vi "esdaq_init.vi"(0 "esdaqPortInp":refnum<visa-resource-name>) -> (1 "esdaqPortOut":refnum<visa-resource-name>, 2 "esdaqErrorOut":errorcluster)   [LabVIEW 2019]
uses:
  <vilib>/Instr/_visa.llb/VISA Flush IO Buffer Mask.ctl
  <vilib>/Instr/_visa.llb/VISA Configure Serial Port (Instr).vi
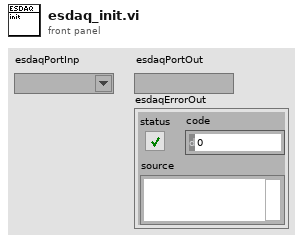
[diagram p1: front panel]
types:
  T1 = typedef "VISA Flush IO Buffer Mask.ctl" = u16
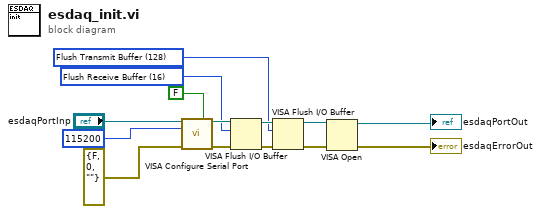
[diagram p0: block diagram]
diagram:
  w6 = T1 128 items=["Flush Receive Buffer"=16, "Write Transmit Buffer to Device"=32, "Flush Receive Buffer (No I/O)"=64, "Flush Transmit Buffer"=128] ("Mask")
  w9 = T1 16 items=["Flush Receive Buffer"=16, "Write Transmit Buffer to Device"=32, "Flush Receive Buffer (No I/O)"=64, "Flush Transmit Buffer"=128] ("Mask")
  n1 = call-poly "VISA Configure Serial Port"("VISA resource name"="esdaqPortInp", "Enable Termination\nChar (T)"=FALSE ("Enable Termination\nChar (T)"), "baud rate (9600)"=u32 115200, "error in (no error)"=errorcluster {"status"=FALSE, "code"=0, "source"=""}) -> ("VISA resource name out"=w10:refnum<visa-resource-name>, "error out"=w11:errorcluster)  [unwired: 10 in]
  n2 = VISA Flush I/O Buffer(VISA resource name=w10, mask (16)=w9, error in (no error)=w11) -> (VISA resource name out=w7:refnum<visa-resource-name>, error out=w8:errorcluster)
  n3 = VISA Flush I/O Buffer(VISA resource name=w7, mask (16)=w6, error in (no error)=w8) -> (VISA resource name out=w3:refnum<visa-resource-name>, error out=w4:errorcluster)
  n4 = VISA Open(error in (no error)=w4, VISA resource name=w3) -> (VISA resource name=→"esdaqPortOut":refnum<visa-resource-name>, error out=→"esdaqErrorOut":errorcluster)  [unwired: 3 in]
